vi "CS-4 Self-Test.vi"(8 "error in (no error)":errorcluster, 11 "VISA session":refnum<visa-resource-name>) -> (0 "error out":errorcluster, 1 "Self-Test Response":string, 2 "Self-Test Error":i32, 3 "dup VISA session":refnum<visa-resource-name>)   [LabVIEW 2016]
doc: "This VI causes the instrument to perform a self-test and returns the results. A numeric indicator indicates if the instrument passed all self-tests, and a string indicator contains the instrument's reponse. If a self test is not supported, the VI returns a warning code."
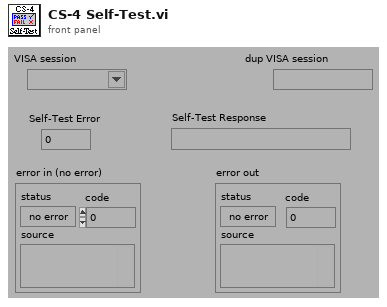
[diagram p1: front panel]
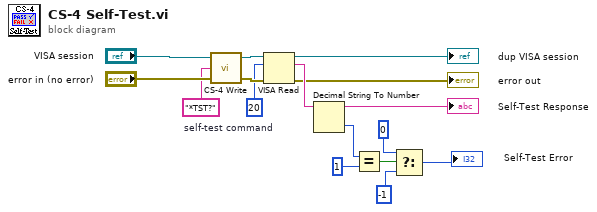
[diagram p0: block diagram]
diagram:
  w10 = "*TST?"  # self-test command
  n1 = call "CS-4 Write.vi"("error in (no error)"="error in (no error)", "write buffer (\"\")"=w10, "VISA session"="VISA session") -> ("error out"=w9:errorcluster, "dup VISA session"=w7:refnum<visa-resource-name>)  [unwired: 1 out]
  n2 = VISA Read(VISA resource name=w7, byte count=u32 20, error in (no error)=w9) -> (VISA resource name out=→"dup VISA session":refnum<visa-resource-name>, read buffer=w15:string, error out=→"error out":errorcluster)  [unwired: 1 out]
  "Self-Test Response" <- w15
  n3 = Decimal String To Number(string=w15) -> (number=w6:i32)  [unwired: 2 in, 1 out]
  n4 = Equal?(x=w6, y=1) -> (x = y?=w4:bool)
  n5 = Select(t=0, s=w4, f=-1) -> (s? t:f=→"Self-Test Error":i32)
